vi "Get DefinedName Identifier Text and SheetId.vi"(8 "error in":errorcluster, 11 "DefinedName in":refnum<k24>) -> (0 "error out":errorcluster, 1 "Range":string, 2 "Identifier":string, 3 "DefinedName out":refnum<k24>, 5 "Sheet Name":string)   [LabVIEW 2019, in "Open Xml.lvlib"]
uses:
  Open Xml.lvlib
  D:/git/Open-Xml-LabVIEW/Source/DocumentFormat.OpenXml.dll
  DocumentFormat.OpenXml.dll
  D:/git/Open-Xml-LabVIEW/Source/DocumentFormat.OpenXml.Framework.dll
  DocumentFormat.OpenXml.Framework.dll
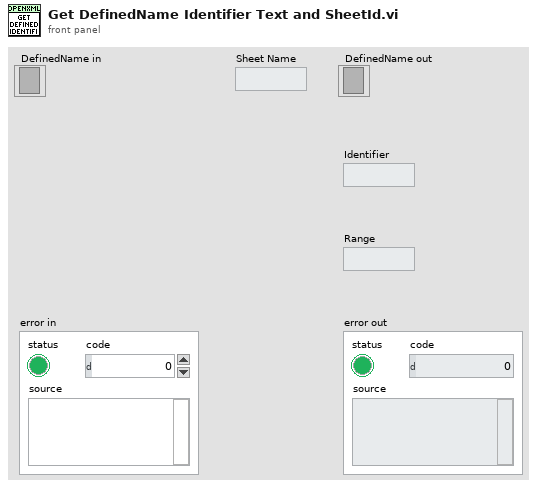
[diagram p1: front panel]
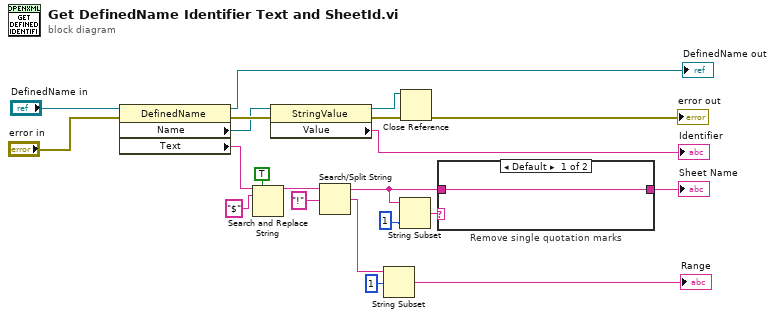
[diagram p0: block diagram]
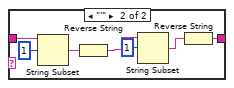
[diagram p2: hidden frame]
diagram:
  n1 = property class="DefinedName"(reference="DefinedName in", error in="error in") -> (reference out=→"DefinedName out":refnum<k24>, error out=w14:errorcluster, "Name"=w10:refnum<k24>, "Text"=w19:string)
  n2 = Search and Replace String(replace all?=TRUE ("replace all? (F)"), input string=w19, search string="$") -> (result string=w18:string)  [unwired: 5 in, 3 out]
  n3 = property class="StringValue"(reference=w10, error in=w14) -> (reference out=w4:refnum<k24>, error out=w11:errorcluster, "Value"=→"Identifier":string)
  n4 = Search/Split String(string=w18, search string/char (-)="!") -> (substring before match=w6:string, match + rest of string=w2:string)  [unwired: 1 in, 1 out]
  n5 = String Subset(string=w2, offset (0)=1) -> (substring=→"Range":string)  [unwired: 1 in]
  n6 = String Subset(string=w6, length (rest)=1 ("length (rest)")) -> (substring=w21:string)  [unwired: 1 in]
  n7 = Close Reference(reference=w4, error in (no error)=w11) -> (error out=→"error out":errorcluster)
  n8 = case "Remove single quotation marks" shown="Default" w21 {
    tunnel: [w22 w23] -> w9
    tunnel: w6 -> [w22 w29]
    frame Default {
    }
    frame "'" {
      n9 = String Subset(string=w29, offset (0)=1) -> (substring=w27:string)  [unwired: 1 in]
      n10 = Reverse String(1:w27) -> (0:w26:string)
      n11 = String Subset(string=w26, offset (0)=1) -> (substring=w25:string)  [unwired: 1 in]
      n12 = Reverse String(1:w25) -> (0:w23:string)
    }
  }
  "Sheet Name" <- w9
